vi "SP_OpCodes.vi"(3 "Commands":string[](array[string])) -> (1 "Commands Out":string[](array[string]))   [LabVIEW 2009]
panel:
  # "This LabVIEW item is deprecated.\n\nIt is believed to be unused and will be removed in a future version of SRV."
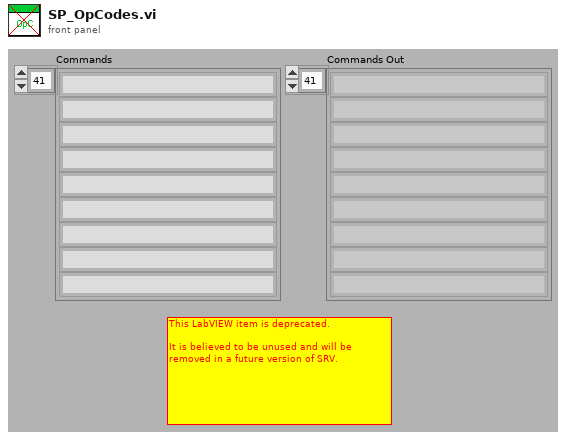
[diagram p1: front panel]
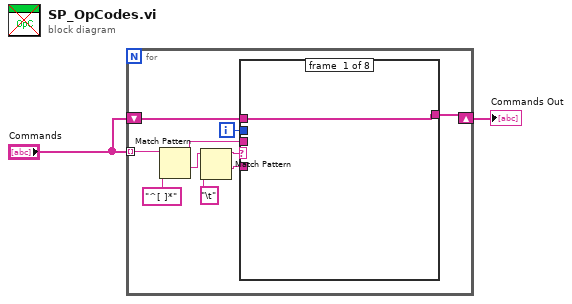
[diagram p0: block diagram]
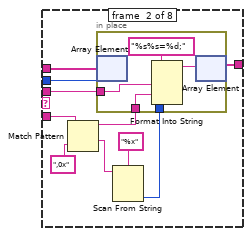
[diagram p2: hidden frame]
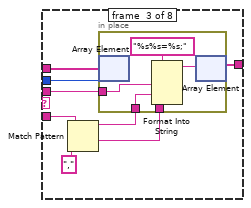
[diagram p3: hidden frame]
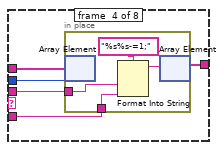
[diagram p4: hidden frame]
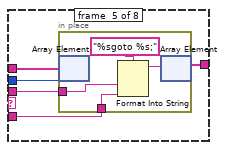
[diagram p5: hidden frame]
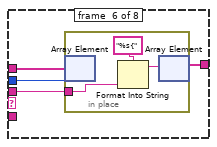
[diagram p6: hidden frame]
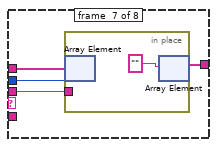
[diagram p7: hidden frame]
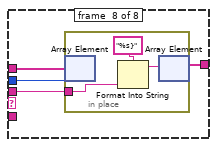
[diagram p8: hidden frame]
diagram:
  n1 = for {
    tunnel: "Commands" -> [w6] mode=indexing
    shift-right: [w8] -> w1
    shift-left: "Commands" -> [w10]
    i -> [w9]
    n2 = Match Pattern(string=w6, regular expression="^[ ]*") -> (match substring=w3:string, after substring=w5:string)  [unwired: 1 in, 2 out]
    n3 = Match Pattern(string=w5, regular expression="\t") -> (before substring=w7:string, after substring=w11:string)  [unwired: 1 in, 2 out]
    n4 = case shown="\"HALTME\"" w7 {
      tunnel: w11 -> [_ w20 w33 w42 w51 _ _ _]
      tunnel: w10 -> [w13 w23 w36 w46 w55 w63 w70 w75]
      tunnel: w9 -> [_ w22 w35 w45 w54 w62 w69 w74]
      tunnel: [w13 w21 w34 w44 w53 w61 w68 w73] -> w8
      tunnel: w3 -> [_ w16 w29 w43 w52 w60 w67 w72]
      frame #0 {
      }
      frame #1 {
        n5 = Match Pattern(string=w20, regular expression=",0x") -> (before substring=w18:string, after substring=w17:string)  [unwired: 1 in, 2 out]
        n6 = Scan From String(format string="%x", input string=w17) -> (output 1=w14:i32)  [unwired: 3 in, 3 out]
        n7 = in-place {
          in-place-border: w18 -> [w26]
          in-place-border: w14 -> [w25]
          in-place-border: w16 -> [w24]
          n8 = in-place-array #1(w23, w22) -> ()  [unwired: 1 out]
          n9 = Format Into String(format string="%s%s=%d;", w24, w26, w25) -> (resulting string=w27:string)  [unwired: 2 in, 1 out]
          n10 = in-place-array #1(w27) -> (w21:string[])  [unwired: 1 out]
        }
      }
      frame #2 {
        n11 = Match Pattern(string=w33, regular expression=",") -> (before substring=w31:string, after substring=w30:string)  [unwired: 1 in, 2 out]
        n12 = in-place {
          in-place-border: w31 -> [w39]
          in-place-border: w30 -> [w38]
          in-place-border: w29 -> [w37]
          n13 = in-place-array #2(w36, w35) -> ()  [unwired: 1 out]
          n14 = Format Into String(format string="%s%s=%s;", w37, w39, w38) -> (resulting string=w40:string)  [unwired: 2 in, 1 out]
          n15 = in-place-array #2(w40) -> (w34:string[])  [unwired: 1 out]
        }
      }
      frame #3 {
        n16 = in-place {
          in-place-border: w42 -> [w48]
          in-place-border: w43 -> [w47]
          n17 = in-place-array #3(w46, w45) -> ()  [unwired: 1 out]
          n18 = Format Into String(format string="%s%s-=1;", w47, w48) -> (resulting string=w49:string)  [unwired: 2 in, 1 out]
          n19 = in-place-array #3(w49) -> (w44:string[])  [unwired: 1 out]
        }
      }
      frame #4 {
        n20 = in-place {
          in-place-border: w51 -> [w57]
          in-place-border: w52 -> [w56]
          n21 = in-place-array #4(w55, w54) -> ()  [unwired: 1 out]
          n22 = Format Into String(format string="%sgoto %s;", w56, w57) -> (resulting string=w58:string)  [unwired: 2 in, 1 out]
          n23 = in-place-array #4(w58) -> (w53:string[])  [unwired: 1 out]
        }
      }
      frame #5 {
        n24 = in-place {
          in-place-border: w60 -> [w64]
          n25 = in-place-array #5(w63, w62) -> ()  [unwired: 1 out]
          n26 = Format Into String(format string="%s{", w64) -> (resulting string=w65:string)  [unwired: 2 in, 1 out]
          n27 = in-place-array #5(w65) -> (w61:string[])  [unwired: 1 out]
        }
      }
      frame #6 {
        n28 = in-place {
          in-place-border: w67 -> [_]
          n29 = in-place-array #6(w70, w69) -> ()  [unwired: 1 out]
          n30 = in-place-array #6("" ("format string")) -> (w68:string[])  [unwired: 1 out]
        }
      }
      frame #7 {
        n31 = in-place {
          in-place-border: w72 -> [w76]
          n32 = in-place-array #7(w75, w74) -> ()  [unwired: 1 out]
          n33 = Format Into String(format string="%s}", w76) -> (resulting string=w77:string)  [unwired: 2 in, 1 out]
          n34 = in-place-array #7(w77) -> (w73:string[])  [unwired: 1 out]
        }
      }
    }
  }
  "Commands Out" <- w1
